vi "Script VIs.vi"(6 "VI Refs":T3, 8 "error in":errorcluster, 9 "Terminal Attributes (Read Msg Output)":T1, 10 "Terminal Attributes (Init Msg Input)":T1) -> (0 "error out":errorcluster)   [LabVIEW 2025, in "_Rescript.lvlib" / "Msg.lvlib" / "Msg.lvclass"]
uses:
  _Rescript/_Rescript.lvclass/_Rescript.ctl
  Msg.lvclass
  Msg.lvclass/Msg.ctl
  <vilib>/Utility/traverseref.llb/TRef TravTarget.ctl
  _Rescript.lvlib
  Name.ctl
  Attributes.ctl
  Terminal Attributes.ctl
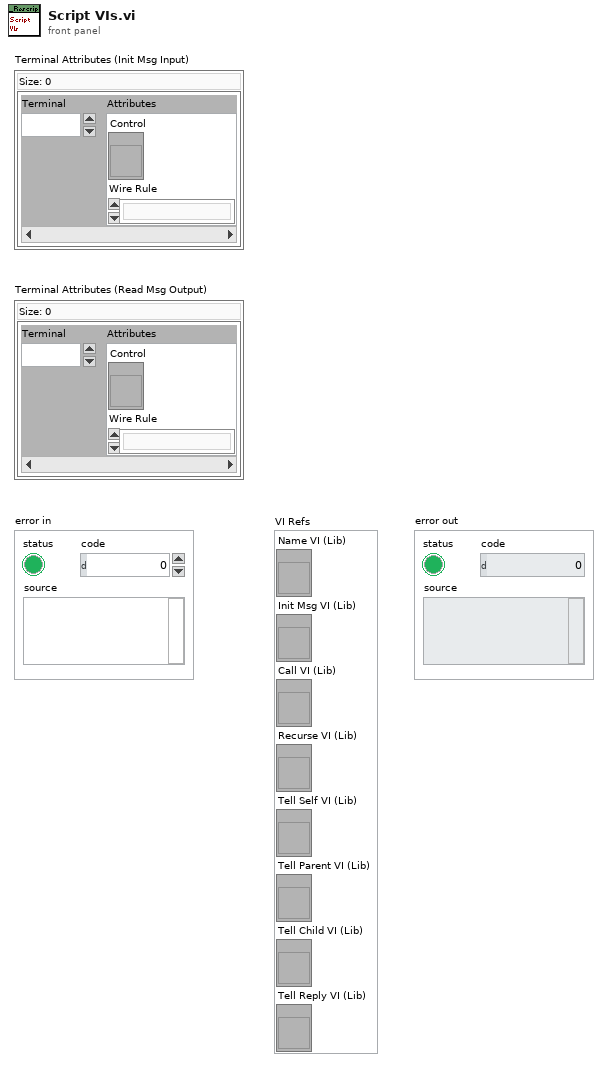
[diagram p1: front panel]
types:
  T1 = typedef "_Rescript.lvlib/Terminal Attributes.ctl" = map{i32, T2}
  T2 = typedef "_Rescript.lvlib/Attributes.ctl" = cluster{"Control":refnum<vi>, "Wire Rule":enum16{"Invalid Wire Rule", "Required", "Recommended", "Optional", "Dynamic Dispatch"}}
  T3 = typedef "_Rescript.lvlib/Msg.lvlib/Msg.lvclass/Name.ctl" = cluster{"Name VI (Lib)":refnum<vi>, "Init Msg VI (Lib)":refnum<vi>, "Call VI (Lib)":refnum<vi>, "Recurse VI (Lib)":refnum<vi>, "Tell Self VI (Lib)":refnum<vi>, "Tell Parent VI (Lib)":refnum<vi>, "Tell Child VI (Lib)":refnum<vi>, "Tell Reply VI (Lib)":refnum<vi>}
  T4 = typedef "TRef TravTarget.ctl" = enum16{"FP", "BD", "Other"}
  T5 = enum16{"Invalid Wire Rule", "Required", "Recommended", "Optional", "Dynamic Dispatch"}
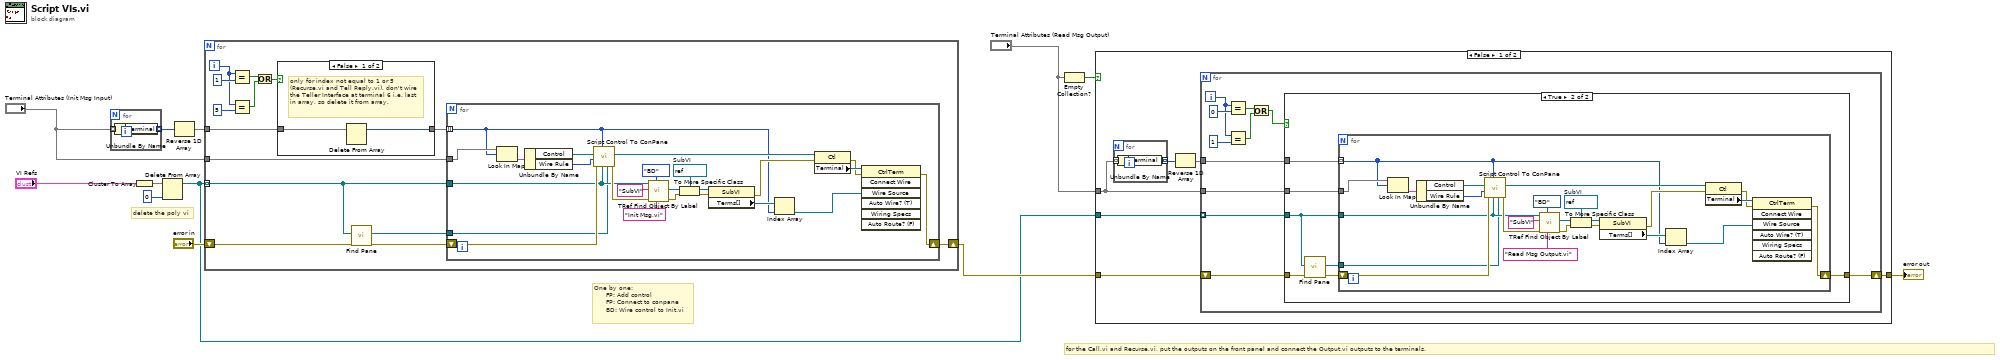
[diagram p0: block diagram]
diagram:
  # "delete the poly vi"
  # "for the Call.vi and Recurse.vi, put the outputs on the front panel and connect the Output.vi outputs to the terminals."
  # "One by one:\n      FP: Add control\n      FP: Connect to conpane\n      BD: Wire control to Init.vi"
  n1 = for {
    tunnel: "Terminal Attributes (Init Msg Input)" -> [w14] mode=indexing
    tunnel: [w13] -> w12 mode=indexing
    n2 = Unbundle By Name(w14) -> ("Terminal"=w13:i32)
  }
  n3 = Cluster To Array(cluster="VI Refs") -> (array=w4:refnum<vi>[])
  n4 = Delete From Array(array=w4, index=0) -> (array with subset deleted=w3:refnum<vi>[])  [unwired: 1 in, 1 out]
  n5 = Reverse 1D Array(array=w12) -> (reversed array=w11:i32[])
  n6 = for {
    tunnel: w11 -> [w25]
    tunnel: "Terminal Attributes (Init Msg Input)" -> [w28]
    shift-right: [w27] -> w7
    shift-left: "error in" -> [w17]
    tunnel: w3 -> [w15] mode=indexing
    i -> [w19]
    n7 = Equal?(x=w19, y=1) -> (x = y?=w23:bool)
    n8 = Equal?(x=w19, y=5) -> (x = y?=w20:bool)
    n9 = Or(x=w23, y=w20) -> (x .or. y?=w22:bool)
    n10 = case shown="False" w22 {
      tunnel: w25 -> [w30 w31]
      tunnel: [w29 w31] -> w24
      frame False {
        # "only for index not equal to 1 or 5 (Recurse.vi and Tell Reply.vi), don't wire the Teller Interface at terminal 6 i.e. last in array, so delete it from array."
        n11 = Delete From Array(array=w30) -> (array with subset deleted=w29:i32[])  [unwired: 2 in, 1 out]
      }
      frame True {
      }
    }
    n12 = call "Find Pane.vi"("error in"=w17, "VI Ref"=w15) -> ("error out"=w18:errorcluster, "Pane Ref"=w16:refnum<vi>)  [unwired: 8 in]
    n13 = for {
      tunnel: w24 -> [w32] mode=indexing
      tunnel: w28 -> [w35]
      tunnel: w16 -> [w37]
      tunnel: w15 -> [w38]
      shift-right: [w53] -> w27
      shift-left: w18 -> [w41]
      w51 = refnum<vi> refnum  # SubVI
      n14 = Look In Map(map=w35, key=w32) -> (value=w36:T2)  [unwired: 1 in, 1 out]
      n15 = Unbundle By Name(w36) -> ("Control"=w34:refnum<vi>, "Wire Rule"=w33:T5)
      n16 = call "Script Control To ConPane.vi"("Pane"=w37, "VI Ref"=w38, "Terminal Index"=w32, "error in"=w41, "Wire Rule"=w33, "Control To Duplicate"=w34) -> ("error out"=w40:errorcluster, "Duplicated Control"=w39:refnum<vi>)  [unwired: 4 in]
      n17 = call <vilib>:"TRef Find Object By Label.vi"("Label"="Init Msg.vi", "Traverse Target"=TRef_TravTarget."BD", "error in (no error)"=w40, "Class Name"="SubVI", "VI Ref"=w38) -> ("error out"=w50:errorcluster, "Found Obj Ref"=w45:refnum<vi>)  [unwired: 3 in, 2 out]
      n18 = To More Specific Class(target class=w51, reference=w45, error in=w50) -> (specific class reference=w48:refnum<vi>, error out=w47:errorcluster)
      n19 = property class="SubVI"(reference=w48, error in=w47) -> (error out=w42:errorcluster, "Terms[]"=w46:refnum<vi>[])  [unwired: 1 out]
      n20 = Index Array(array=w46, index=w32) -> (element=w43:refnum<vi>)
      n21 = property class="Ctl"(reference=w39, error in=w42) -> (error out=w54:errorcluster, "Terminal"=w55:refnum<vi>)  [unwired: 1 out]
      n22 = invoke class="CtrlTerm" method="Connect Wire"(reference=w55, error in=w54, "Wire Source"=w43) -> (error out=w53:errorcluster)  [unwired: 4 in, 6 out]
    }
  }
  n23 = Empty Collection?(1:"Terminal Attributes (Read Msg Output)") -> (0:w8:bool)
  n24 = case shown="False" w8 {
    tunnel: w3 -> [w61 _]
    tunnel: "Terminal Attributes (Read Msg Output)" -> [w59 _]
    tunnel: w7 -> [w57 w107]
    tunnel: [w56 w107] -> w6
    frame False {
      n25 = for {
        tunnel: w59 -> [w63] mode=indexing
        tunnel: [w62] -> w60 mode=indexing
        n26 = Unbundle By Name(w63) -> ("Terminal"=w62:i32)
      }
      n27 = Reverse 1D Array(array=w60) -> (reversed array=w58:i32[])
      n28 = for {
        tunnel: w58 -> [w65]
        tunnel: w59 -> [w74]
        shift-right: [w72] -> w56
        shift-left: w57 -> [w73]
        tunnel: w61 -> [w70] mode=indexing
        i -> [w66]
        n29 = Equal?(x=w66, y=0) -> (x = y?=w69:bool)
        n30 = Equal?(x=w66, y=1) -> (x = y?=w67:bool)
        n31 = Or(x=w69, y=w67) -> (x .or. y?=w64:bool)
        n32 = case shown="True" w64 {
          tunnel: w74 -> [_ w82]
          tunnel: w73 -> [w75 w76]
          tunnel: [w75 w81] -> w72
          tunnel: w70 -> [_ w79]
          tunnel: w65 -> [_ w80]
          frame False {
          }
          frame True {
            n33 = call "Find Pane.vi"("error in"=w76, "VI Ref"=w79) -> ("error out"=w77:errorcluster, "Pane Ref"=w78:refnum<vi>)  [unwired: 8 in]
            n34 = for {
              tunnel: w80 -> [w83] mode=indexing
              tunnel: w82 -> [w86]
              tunnel: w78 -> [w88]
              tunnel: w79 -> [w89]
              shift-right: [w104] -> w81
              shift-left: w77 -> [w92]
              w102 = refnum<vi> refnum  # SubVI
              n35 = Look In Map(map=w86, key=w83) -> (value=w87:T2)  [unwired: 1 in, 1 out]
              n36 = Unbundle By Name(w87) -> ("Control"=w85:refnum<vi>, "Wire Rule"=w84:T5)
              n37 = call "Script Control To ConPane.vi"("Pane"=w88, "VI Ref"=w89, "Terminal Index"=w83, "error in"=w92, "Wire Rule"=w84, "Control To Duplicate"=w85) -> ("error out"=w91:errorcluster, "Duplicated Control"=w90:refnum<vi>)  [unwired: 4 in]
              n38 = call <vilib>:"TRef Find Object By Label.vi"("Label"="Read Msg Output.vi", "Traverse Target"=TRef_TravTarget."BD", "error in (no error)"=w91, "Class Name"="SubVI", "VI Ref"=w89) -> ("error out"=w101:errorcluster, "Found Obj Ref"=w96:refnum<vi>)  [unwired: 3 in, 2 out]
              n39 = To More Specific Class(target class=w102, reference=w96, error in=w101) -> (specific class reference=w99:refnum<vi>, error out=w98:errorcluster)
              n40 = property class="SubVI"(reference=w99, error in=w98) -> (error out=w93:errorcluster, "Terms[]"=w97:refnum<vi>[])  [unwired: 1 out]
              n41 = Index Array(array=w97, index=w83) -> (element=w94:refnum<vi>)
              n42 = property class="Ctl"(reference=w90, error in=w93) -> (error out=w105:errorcluster, "Terminal"=w106:refnum<vi>)  [unwired: 1 out]
              n43 = invoke class="CtrlTerm" method="Connect Wire"(reference=w106, error in=w105, "Wire Source"=w94) -> (error out=w104:errorcluster)  [unwired: 4 in, 6 out]
            }
          }
        }
      }
    }
    frame True {
    }
  }
  "error out" <- w6
